vi "XY Graph Save Plot.vi"(6 "Delimiter (TAB)":string="\t", 8 "Error In":errorcluster, 9 "Plot Index":i32, 11 "XYGraph Ref":T1) -> (0 "Error Out":errorcluster, 1 "File Path":path, 2 "Plot Name":string, 3 "XYGraph Ref":T1, 5 "Graph Caption":string)   [LabVIEW 2019, in "XY Graph Add-Ons.lvlib"]
uses:
  XY Graph Add-Ons.lvlib
  XY Graph Refnum.ctl
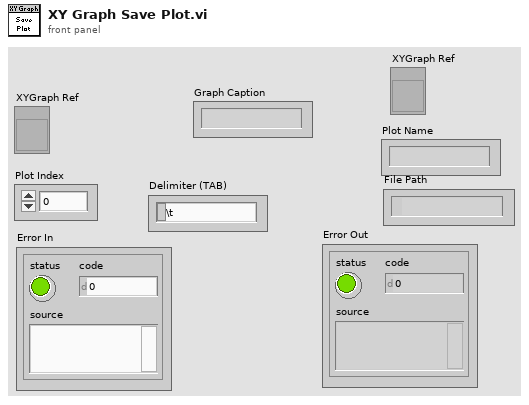
[diagram p1: front panel]
types:
  T1 = typedef "XY Graph Add-Ons.lvlib/XY Graph Refnum.ctl" = refnum<vi>
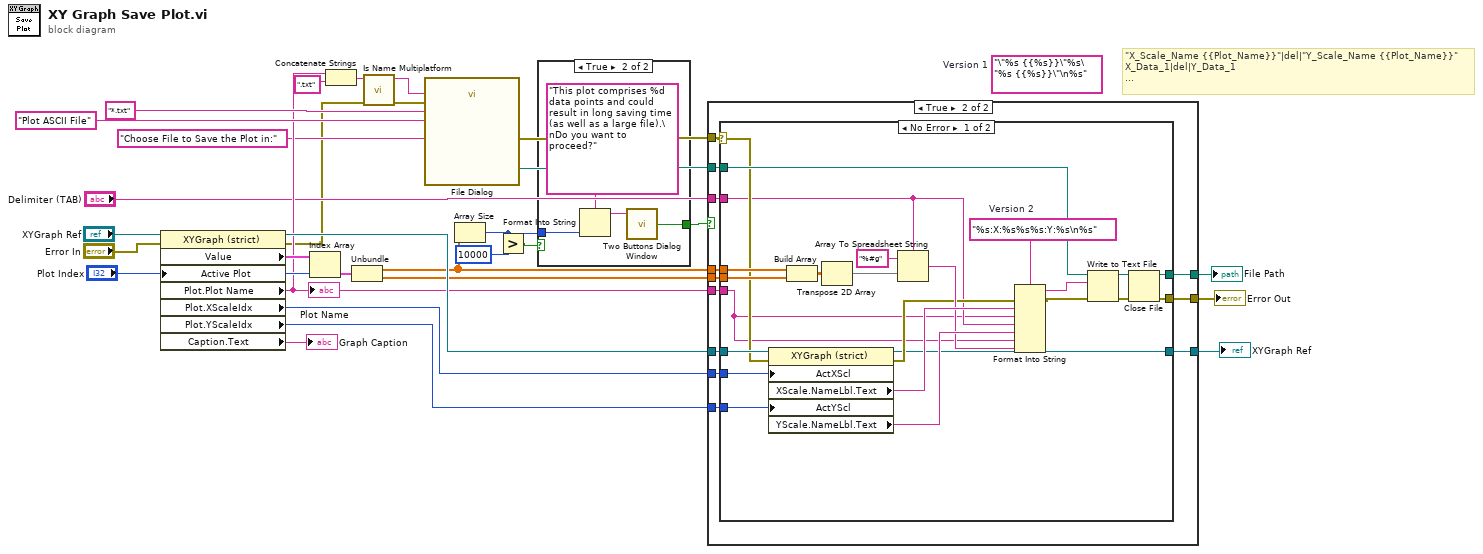
[diagram p0: block diagram]
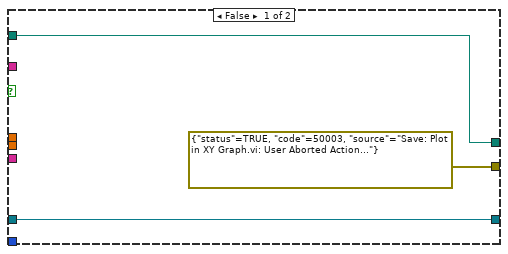
[diagram p2: hidden frame]
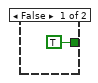
[diagram p4: hidden frame]
diagram:
  (unwired) "\"%s {{%s}}\"%s\"%s {{%s}}\"\n%s"  # Version 1
  # "\"X_Scale_Name {{Plot_Name}}\"|del|\"Y_Scale_Name {{Plot_Name}}\"\nX_Data_1|del|Y_Data_1\n..."
  n1 = property class="XYGraph (strict)"(reference="XYGraph Ref", error in="Error In", "Active Plot"="Plot Index") -> (reference out=w26:T1, error out=w3:errorcluster, "Value"=w29:cluster{"X Array":dbl[], "Y Array":dbl[]}[], "Plot.Plot Name"=w20:string, "Plot.XScaleIdx"=w25:u32, "Plot.YScaleIdx"=w24:u32, "Caption.Text"=→"Graph Caption":string)
  "Plot Name" <- w20
  n2 = Index Array(array=w29, index="Plot Index") -> (element=w27:cluster{"X Array":dbl[], "Y Array":dbl[]})
  n3 = Concatenate Strings(w20, ".txt" ("string")) -> (w12:string)
  n4 = Unbundle(w27) -> ("X Array"=w8:dbl[], "Y Array"=w23:dbl[])
  n5 = call <vilib>:"Is Name Multiplatform.vi"("error in (no error)"=w3, "filename"=w12) -> ("error out"=w10:errorcluster, "suggested filename"=w9:string)  [unwired: 5 in, 3 out]
  n6 = call "File Dialog"("prompt"="Choose File to Save the Plot in:", "default name"=w9, "error in"=w10, "pattern (all files)"="*.txt", "pattern label"="Plot ASCII File") -> ("selected path"=w18:path, "error out"=w15:errorcluster)  [unwired: 7 in, 2 out]
  n7 = Array Size(array=w8) -> (size(s)=w6:i32)
  n8 = Greater?(x=w6, y=10000) -> (0:w5:bool)
  n9 = case shown="True" w5 {
    tunnel: w6 -> [_ w34]
    tunnel: [TRUE ("T button?") w32] -> w4
    frame False {
    }
    frame True {
      n10 = Format Into String(format string="This plot comprises %d data points and could result in long saving time (as well as a large file).\nDo you want to proceed?", w34) -> (resulting string=w33:string)  [unwired: 2 in, 1 out]
      n11 = call "Two Buttons Dialog Window.vi"("Message"=w33) -> ("OK?"=w32:bool)  [unwired: 2 in]
    }
  }
  n12 = case shown="True" w4 {
    tunnel: w26 -> [w36 w50]
    tunnel: w25 -> [_ w49]
    tunnel: w24 -> [_ w48]
    tunnel: w23 -> [_ w47]
    tunnel: w20 -> [_ w46]
    tunnel: w18 -> [w37 w45]
    tunnel: [errorcluster {"status"=TRUE, "code"=50003, "source"="Save: Plot in XY Graph.vi: User Aborted Action..."} ("error IO") w44] -> w17
    tunnel: [w37 w43] -> w16
    tunnel: w15 -> [_ w42]
    tunnel: "Delimiter (TAB)" -> [_ w41]
    tunnel: w8 -> [_ w40]
    tunnel: [w36 w39] -> w1
    frame False {
    }
    frame True {
      n13 = case shown="No Error" w42 {
        selector: w42 -> [w56 w76]
        tunnel: w50 -> [w74 w75]
        tunnel: w49 -> [w73 _]
        tunnel: w48 -> [w72 _]
        tunnel: w40 -> [w71 _]
        tunnel: w47 -> [w70 _]
        tunnel: w46 -> [w53 _]
        tunnel: w45 -> [w60 _]
        tunnel: [w54 w76] -> w44
        tunnel: [w52 _] -> w43
        tunnel: w41 -> [w55 _]
        tunnel: [w51 w75] -> w39
        frame No Error {
          w66 = "%s:X:%s%s%s:Y:%s\n%s"  # Version 2
          n14 = property class="XYGraph (strict)"(reference=w74, error in=w56, "ActXScl"=w73, "ActYScl"=w72) -> (reference out=w51:T1, error out=w62:errorcluster, "XScale.NameLbl.Text"=w65:string, "YScale.NameLbl.Text"=w64:string)
          n15 = Build Array(w71, w70) -> (w69:dbl[][])
          n16 = Transpose 2D Array(2D array=w69) -> (transposed array=w68:dbl[][])
          n17 = Array To Spreadsheet String(delimiter (Tab)=w55, array=w68, 3:"%#g" ("format string")) -> (spreadsheet string=w63:string)
          n18 = Format Into String(format string=w66, error in=w62, w65, w53, w55, w64, w53, w63) -> (resulting string=w61:string, error out=w59:errorcluster)  [unwired: 1 in]
          n19 = Write to Text File(file (use dialog)=w60, text=w61, error in=w59) -> (refnum out=w58:refnum<file>, error out=w57:errorcluster)  [unwired: 1 in, 1 out]
          n20 = Close File(refnum=w58, error in=w57) -> (path=w52:path, error out=w54:errorcluster)
        }
        frame Error {
        }
      }
    }
  }
  "Error Out" <- w17
  "File Path" <- w16
  "XYGraph Ref" <- w1
